vi "polytoroi.vi"(11 "Rectangle Points 2":T1[](array[typedef])=[{"X"=194.0, "Y"=132.0}, {"X"=460.0, "Y"=60.0}, {"X"=493.0, "Y"=182.0}, {"X"=227.0, "Y"=254.0}, {"X"=194.0, "Y"=132.0}] {"Y" format="%.2f"; "X" format="%.2f"}) -> (3 "ROI Descriptor 4":T2 {"Contours"."Type" items=["No Selection", "Point", "Line", "Rectangle", "Oval", "Polygon", "Freehand Region", "Annulus", "Unused2", "Unused3", "Broken Line", "Freehand Line", "Rotated Rectangle"]})   [LabVIEW 2015]
panel:
  out "R":dbl
  out "d":dbl
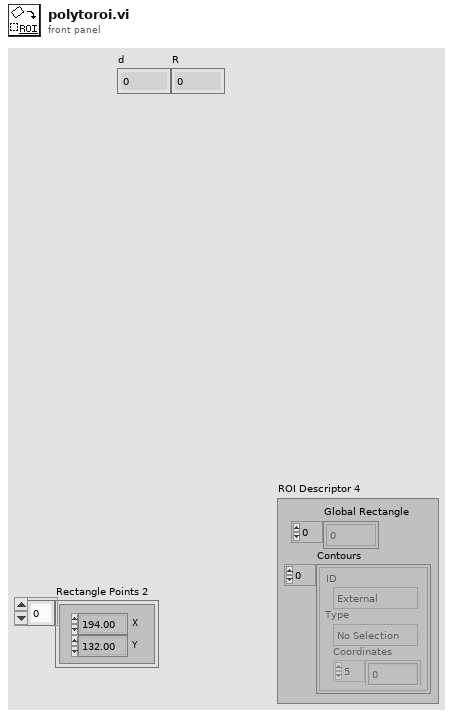
[diagram p1: front panel]
types:
  T1 = typedef "IMAQ Point" = cluster{"X":sgl, "Y":sgl}
  T2 = typedef "ROI Descriptor" = cluster{"Global Rectangle":i32[], "Contours":cluster{"ID":enum32{"External", "Internal"}, "Type":u32, "Coordinates":i32[]}[]}
  T3 = cluster{"ID":enum32{"External", "Internal"}, "Type":u32, dbl[]}
  T4 = cluster{"ID":enum32{"External", "Internal"}, "Type":u32, dbl[]}[]
  T5 = cluster{i32[], cluster{"ID":enum32{"External", "Internal"}, "Type":u32, dbl[]}[]}
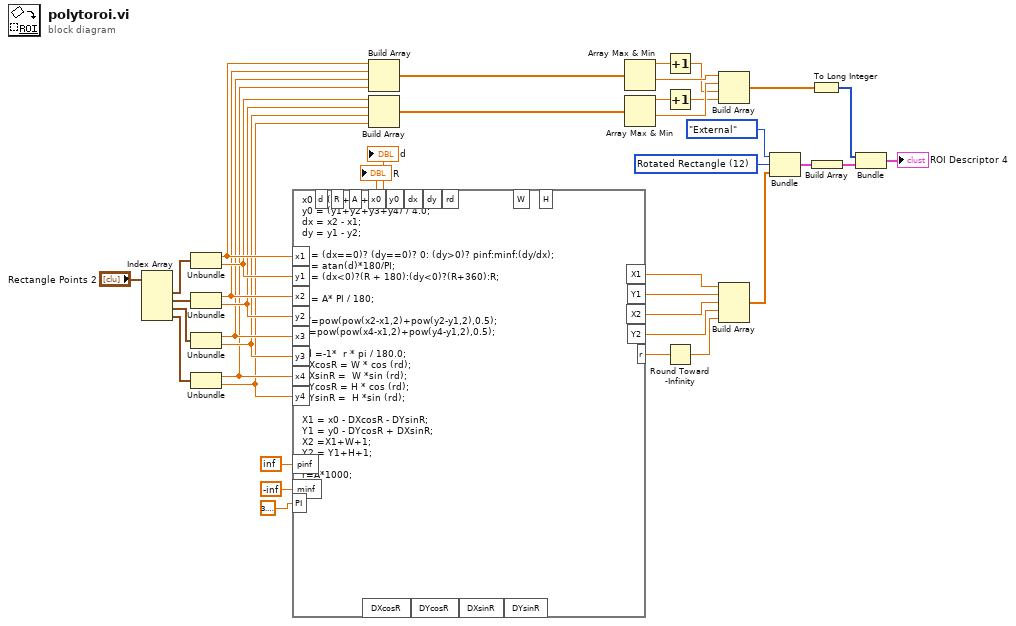
[diagram p0: block diagram]
diagram:
  w26 = u32 12 items=["No Selection", "Point", "Line", "Rectangle", "Oval", "Polygon", "Freehand Region", "Annulus", "Unused2", "Unused3", "Broken Line", "Freehand Line", "Rotated Rectangle"] ("Type")
  n1 = Index Array(array="Rectangle Points 2") -> (element #1=w39:T1, element #2=w38:T1, element #3=w37:T1, element #4=w36:T1)  [unwired: 4 in]
  n2 = Unbundle(w39) -> ("X"=w18:sgl, "Y"=w17:sgl)
  n3 = Unbundle(w38) -> ("X"=w16:sgl, "Y"=w15:sgl)
  n4 = Unbundle(w37) -> ("X"=w14:sgl, "Y"=w13:sgl)
  n5 = Unbundle(w36) -> ("X"=w12:sgl, "Y"=w11:sgl)
  n6 = formula code="x0 = (x1+x2+x3+x4) / 4.0;\ny0 = (y1+y2+y3+y4) / 4.0;\ndx = x2 - x1;\ndy = y1 - y2;\n\nd = (dx==0)? (dy==0)? 0: (dy>0)? pinf:minf:(dy/dx);\nR = atan(d)*180/PI;\nA = (dx<0)?(R + 180):(dy<0)?(R+360):R;\n\nR = A* PI / 180;\n\nW=pow(pow(x2-x1,2)+pow(y2-y1,2),0.5);\nH=pow(pow(x4-x1,2)+pow(y4-y1,2),0.5);\n\nrd =-1*  r * pi / 180.0;\nDXcosR = W * cos (rd);\nDXsinR =  W *sin (rd);\nDYcosR = H * cos (rd);\nDYsinR =  H *sin (rd);\n\nX1 = x0 - DXcosR - DYsinR;\nY1 = y0 - DYcosR + DXsinR;\nX2 =X1+W+1;\nY2 = Y1+H+1;\n\nr=A*1000;"("x1"=w18, "y1"=w17, "x2"=w16, "y2"=w15, "x3"=w14, "y3"=w13, "x4"=w12, "y4"=w11, "pinf"=inf, "minf"=-inf, "PI"=3.141592653589793) -> ("X1"=w7:dbl, "Y1"=w6:dbl, "X2"=w5:dbl, "Y2"=w4:dbl, "r"=w3:dbl, "d"=→"d":dbl, "R"=→"R":dbl)  [unwired: 12 out]
  n7 = Build Array(w18, w16, w14, w12) -> (w35:sgl[])
  n8 = Build Array(w17, w15, w13, w11) -> (w34:sgl[])
  n9 = Array Max & Min(array=w35) -> (max value=w22:sgl, min value=w33:sgl)  [unwired: 2 out]
  n10 = Array Max & Min(array=w34) -> (max value=w20:sgl, min value=w32:sgl)  [unwired: 2 out]
  n11 = Increment(x=w22) -> (x+1=w21:sgl)
  n12 = Increment(x=w20) -> (x+1=w19:sgl)
  n13 = Round Toward -Infinity(1:w3) -> (0:w24:dbl)
  n14 = Build Array(w33, w32, w21, w19) -> (w31:sgl[])
  n15 = Build Array(w7, w6, w5, w4, w24) -> (w23:dbl[])
  n16 = Bundle("ID"=enum32{"External", "Internal"}."External", "Type"=w26, w23) -> (w28:T3)  [unwired: 1 in]
  n17 = To Long Integer(number=w31) -> (32bit integer=w25:i32[])
  n18 = Build Array(w28) -> (w29:T4)
  n19 = Bundle(w25, w29) -> (→"ROI Descriptor 4":T5)  [unwired: 1 in]
